vi "UNBILITZ-SimulationFunctionalGlobal.vi"(8 "error in (no error)":errorcluster, 9 "VISA Resource Name":string, 10 "Simulation Mode":bool, 11 "Operation (Get)":T1) -> (0 "error out":errorcluster, 3 "Simulation Mode":bool)   [LabVIEW 2011]
doc: "This VI holds the simulation mode state, used in other driver calls to determine whether to write commands to the device or simply pass through in \"simluation mode\"."
uses:
  UNIBLITZ-SimulationModeOperation.ctl
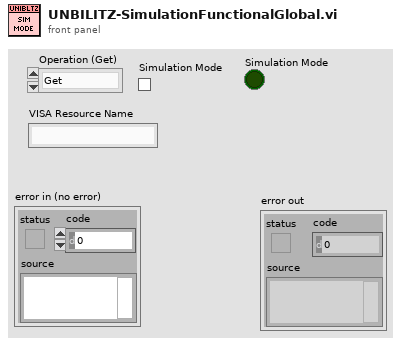
[diagram p1: front panel]
types:
  T1 = typedef "UNIBLITZ-SimulationModeOperation.ctl" = enum16{"Get", "Set"}
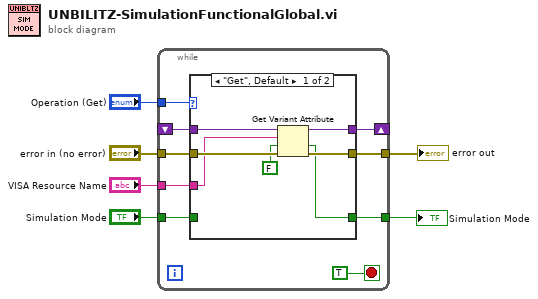
[diagram p0: block diagram]
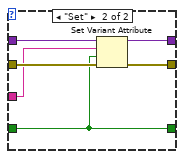
[diagram p2: hidden frame]
diagram:
  n1 = while {
    shift-right: [w14] -> _
    shift-left: _ -> [w13]
    tunnel: "error in (no error)" -> [w12]
    tunnel: [w11] -> w5
    tunnel: [w10] -> w4
    tunnel: "VISA Resource Name" -> [w9]
    tunnel: "Simulation Mode" -> [w8]
    tunnel: "Operation (Get)" -> [w7]
    stop <- TRUE stop-if-true
    n2 = case shown="\"Get\", Default" w7 {
      tunnel: [w19 w28] -> w14
      tunnel: w13 -> [w20 w27]
      tunnel: w12 -> [w22 w26]
      tunnel: [w21 w25] -> w11
      tunnel: w9 -> [w18 w23]
      tunnel: [w16 w24] -> w10
      tunnel: w8 -> [_ w24]
      frame "Get", Default {
        n3 = Get Variant Attribute(Variant=w20, name=w18, default value (empty Variant)=FALSE ("Simulation Mode"), error in=w22) -> (duplicate Variant=w19:variant, value=w16:bool, error out=w21:errorcluster)  [unwired: 1 out]
      }
      frame "Set" {
        n4 = Set Variant Attribute(Variant=w27, name=w23, value=w24, error in=w26) -> (Variant out=w28:variant, error out=w25:errorcluster)  [unwired: 1 out]
      }
    }
  }
  "error out" <- w5
  "Simulation Mode" <- w4
